vi "Version Data.vi"() -> ()   [LabVIEW 2012]
panel:
  in  "Version":string="2.1.0"
  in  "Last Update":timestamp=timestamp(3420814747.2772226 s since 1904-01-01) format="%<%x>T"
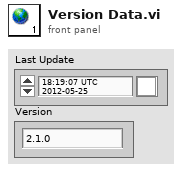
[diagram p1: front panel]
diagram:
